vi "Basic Multitone.vi"(0 "start frequency":dbl=10.0 format="%.2p", 1 "#tones":i32=3, 2 "reset signal":bool, 3 "amplitude":dbl=-1.0 format="%.2p", 7 "seed":i32=-1, 9 "delta frequency":dbl=100.0 format="%.2p", 11 "error in (no error)":errorcluster, 12 "sampling info":cluster{"Fs":dbl, "#s":dbl}={"Fs"=1000.0, "#s"=1000.0} {"Fs" format="%.2p"}, 13 "coerce frequencies?":bool, 14 "phase relationship":u16(ring) items=["random", "linear difference", "linear phase"]) -> (4 "signal out":waveform(dbl), 6 "crest factor":dbl format="%.2p", 10 "actual tone frequencies":dbl[](array[numeric]), 15 "error out":errorcluster)   [LabVIEW 2020, in "NI_MAPro.lvlib"]
doc: "Generates a waveform that is the sum of integer cycle sine tones."
uses:
  NI_MAPro.lvlib
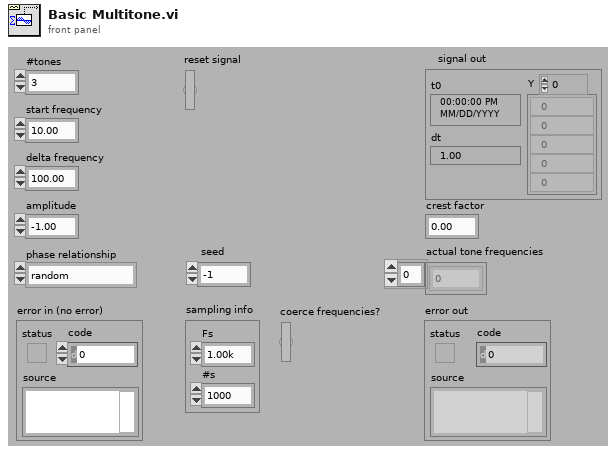
[diagram p1: front panel]
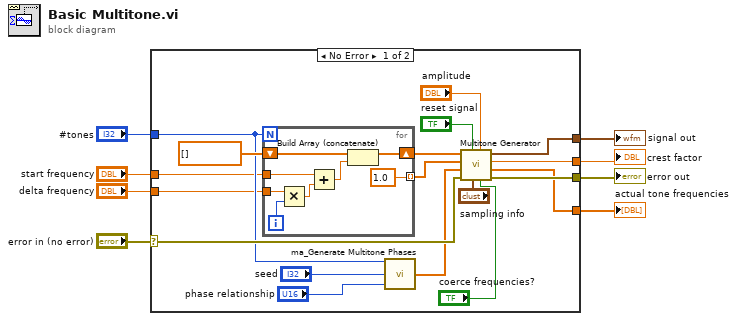
[diagram p0: block diagram]
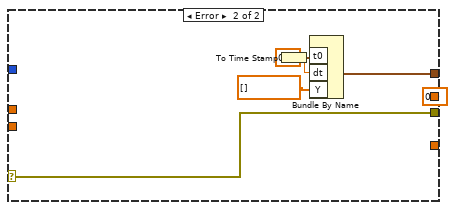
[diagram p2: hidden frame]
diagram:
  n1 = case shown="No Error" "error in (no error)" {
    selector: "error in (no error)" -> [w20 w40]
    tunnel: [w24 w40] -> w8
    tunnel: [w17 0.0 ("crest factor")] -> w6
    tunnel: [w16 w37] -> w5
    tunnel: [w13 _] -> w4
    tunnel: "#tones" -> [w11 _]
    tunnel: "start frequency" -> [w10 _]
    tunnel: "delta frequency" -> [w9 _]
    frame No Error {
      n2 = for {
        N: w11 -> [_]
        shift-right: [w33] -> w25
        shift-left: dbl[] [] -> [w34]
        tunnel: w9 -> [w31]
        tunnel: w10 -> [w30]
        tunnel: [1.0] -> w23 mode=indexing
        i -> [w32]
        n3 = Multiply(x=w31, y=w32) -> (x*y=w29:dbl)
        n4 = Add(x=w30, y=w29) -> (x+y=w28:dbl)
        n5 = Build Array (concatenate)(w34, w28) -> (w33:dbl[])
      }
      n6 = call "ma_Generate Multitone Phases.vi"("phase relationship"="phase relationship", "seed"="seed", "#tones"=w11) -> ("Tone Phases"=w18:dbl[])
      n7 = call "Multitone Generator.vi"("coerce frequencies?"="coerce frequencies?", "amplitude"="amplitude", "sampling info"="sampling info", "reset signal"="reset signal", "error in (no error)"=w20, "tone phases"=w18, "tone amplitudes"=w23, "tone frequencies"=w25) -> ("error out"=w24:errorcluster, "actual tone frequencies"=w13:dbl[], "crest factor"=w17:dbl, "signal out"=w16:waveform(dbl))
    }
    frame Error {
      w39 = 0.0 ("t0")
      n8 = To Time Stamp(1:w39) -> (0:w35:timestamp)
      n9 = Bundle By Name("t0"=w35, "dt"=w39, "Y"=dbl[] []) -> (w37:waveform(dbl))  [unwired: 1 out]
    }
  }
  "error out" <- w8
  "crest factor" <- w6
  "signal out" <- w5
  "actual tone frequencies" <- w4
